vi "Queue Actor.vi"(8 "Queue Caller":map{string, refnum<data-value>}(c390), 9 "Queue of Queue Self":refnum<queue>, 10 "Queue Self Alias":string, 11 "Queue jettl":refnum<class "Queue jettl.lvclass">) -> ()   [LabVIEW 2021, in "jettl.lvlib" / "Base Queue jettl.lvlib" / "Base Queue jettl.lvclass"]
uses:
  Base Queue jettl.lvclass
  Queue jettl/Queue jettl.lvclass
  C:/git/jettl/src/jettl/jettl/jettl/jettl.lvclass
  Msg Strategy/Msg Strategy.lvclass
  C:/git/jettl/src/jettl/jettl/Queue jettl/Queue jettl.lvclass
  Queue Last Ack/Queue Last Ack Msg Strategy/Queue Last Ack Msg Strategy.lvclass
  C:/git/jettl/src/jettl/Msg Strategy/Msg Strategy/Msg Strategy.lvclass
  jettl.lvlib
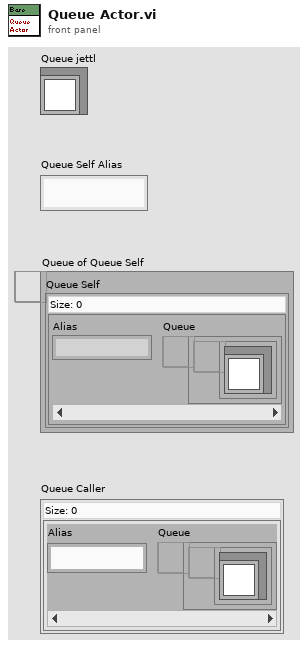
[diagram p1: front panel]
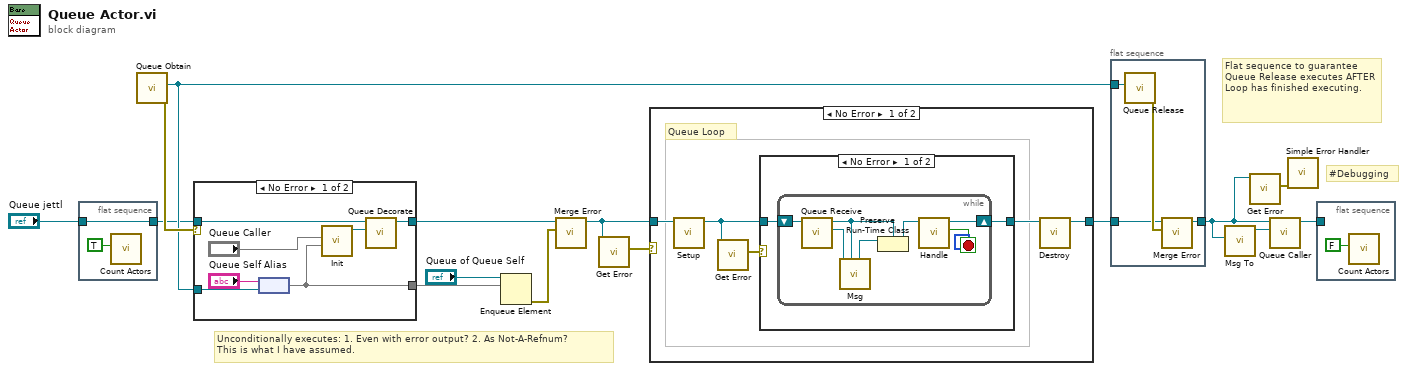
[diagram p0: block diagram]
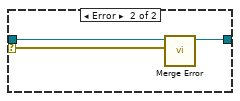
[diagram p2: hidden frame]
diagram:
  # "#Debugging"
  # "Flat sequence to guarantee Queue Release executes AFTER Loop has finished executing."
  # "Unconditionally executes: 1. Even with error output? 2. As Not-A-Refnum?\nThis is what I have assumed."
  n1 = flat-sequence {
    tunnel: [w16] -> w2
    tunnel: "Queue jettl" -> [w16]
    frame #0 {
      n2 = call "Count Actors.vi"("Increment?"=TRUE) -> ()  [unwired: 11 in]
    }
  }
  n3 = call "Queue Obtain.vi"() -> ("error out"=w15:errorcluster, "Queue"=w11:refnum<data-value>)  [unwired: 10 in]
  n4 = case shown="No Error" w15 {
    selector: w15 -> [_ w26]
    tunnel: [w18 w27] -> w10
    tunnel: w2 -> [w24 w25]
    tunnel: w11 -> [w21 _]
    tunnel: [w19 _] -> w9
    frame No Error {
      n5 = node("Queue Self Alias", w21) -> (w19:map{string, refnum<data-value>})
      n6 = call "Init.vi"("Queue Self"=w19, "Queue Caller"="Queue Caller") -> ("Base Queue jettl out"=w23:refnum<class "Base Queue jettl.lvclass">)  [unwired: 9 in]
      n7 = call-dynamic "Queue Decorate.vi"("Queue jettl"=w23, "Queue jettl in"=w24) -> ("Queue jettl out"=w18:refnum<class "Queue jettl.lvclass">)  [unwired: 9 in]
    }
    frame Error {
      n8 = call-dynamic "Merge Error.vi"("Error"=w26, "Merge Error in"=w25) -> ("Merge Error out"=w27:refnum<class "Queue jettl.lvclass">)  [unwired: 9 in]
    }
  }
  n9 = Enqueue Element(queue="Queue of Queue Self", element=w9) -> (error out=w13:errorcluster)  [unwired: 2 in, 2 out]
  n10 = call-dynamic "Merge Error.vi"("Error"=w13, "Merge Error in"=w10) -> ("Merge Error out"=w14:refnum<class "Queue jettl.lvclass">)  [unwired: 9 in]
  n11 = call-dynamic "Get Error.vi"("jettl in"=w14) -> ("Error"=w8:errorcluster)  [unwired: 10 in]
  n12 = case shown="No Error" w8 {
    tunnel: w14 -> [w30 w43]
    tunnel: [w31 w43] -> w7
    frame No Error {
      # "Queue Loop"
      n13 = call-dynamic "Setup.vi"("Setup in"=w30) -> ("Setup out"=w28:refnum<class "Queue jettl.lvclass">)  [unwired: 10 in]
      n14 = call-dynamic "Get Error.vi"("jettl in"=w28) -> ("Error"=w29:errorcluster)  [unwired: 10 in]
      n15 = case shown="No Error" w29 {
        tunnel: [w34 w42] -> w32
        tunnel: w28 -> [w33 w42]
        frame No Error {
          n16 = while "Queue Loop" {
            shift-right: [w41] -> w34
            shift-left: w33 -> [w40]
            stop <- w38 stop-if-true
            n17 = call-dynamic "Queue Receive.vi"("Queue jettl in"=w40) -> ("Msg Strategy"=w39:refnum<class "Msg Strategy.lvclass">, "Queue jettl out"=w37:refnum<class "Queue jettl.lvclass">)  [unwired: 9 in]
            n18 = call-dynamic "Msg.vi"("jettl in"=w37, "Msg Strategy in"=w39) -> ("jettl out"=w35:refnum<class "jettl.lvclass">)  [unwired: 9 in]
            n19 = Preserve Run-Time Class(object in=w35, 2:w37) -> (object out=w36:refnum<class "Queue jettl.lvclass">)  [unwired: 1 in, 1 out]
            n20 = call-dynamic "Handle.vi"("jettl in"=w36) -> ("Destroy?"=w38:bool, "jettl out"=w41:refnum<class "Queue jettl.lvclass">)  [unwired: 9 in]
          }
        }
        frame Error {
        }
      }
      n21 = call-dynamic "Destroy.vi"("jettl in"=w32) -> ("jettl out"=w31:refnum<class "Queue jettl.lvclass">)  [unwired: 10 in]
    }
    frame Error {
    }
  }
  n22 = flat-sequence {
    tunnel: w11 -> [w47]
    tunnel: [w46] -> w4
    tunnel: w7 -> [w44]
    frame #0 {
      n23 = call "Queue Release.vi"("Queue"=w47) -> ("error out"=w45:errorcluster)  [unwired: 10 in]
      n24 = call-dynamic "Merge Error.vi"("Error"=w45, "Merge Error in"=w44) -> ("Merge Error out"=w46:refnum<class "Queue jettl.lvclass">)  [unwired: 9 in]
    }
  }
  n25 = call "Msg To.vi"("Queue jettl"=w4) -> ("Queue Last Ack Msg Strategy out"=w6:refnum<class "Queue Last Ack Msg Strategy.lvclass">)  [unwired: 10 in]
  n26 = call-dynamic "Get Error.vi"("jettl in"=w4) -> ("Error"=w5:errorcluster)  [unwired: 10 in]
  n27 = call-dynamic "Queue Caller.vi"("Msg Strategy"=w6, "jettl in"=w4) -> ("jettl out"=w1:refnum<class "Queue jettl.lvclass">)  [unwired: 9 in]
  n28 = call <vilib>:"Simple Error Handler.vi"("error in (no error)"=w5) -> ()  [unwired: 4 in, 5 out]
  n29 = flat-sequence {
    tunnel: w1 -> [_]
    frame #0 {
      n30 = call "Count Actors.vi"("Increment?"=FALSE) -> ()  [unwired: 11 in]
    }
  }
